vi "collectAI_img.vi"() -> (0 "wrap":i32)   [LabVIEW 2015]
uses:
  <vilib>/DAQmx/read.llb/DAQmx Read (Analog 2D I16 NChan NSamp).vi
  <vilib>/DAQmx/miscellaneous.llb/DAQmx Fill In Error Info.vi
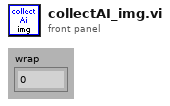
[diagram p1: front panel]
types:
  T1 = typedef "LVRectTypeDef.ctl" = cluster{"Left":i16, "Top":i16, "Right":i16, "Bottom":i16}
  T2 = cluster{"Xpixels":i32, "Vxminref":dbl, "Vxmaxref":dbl, "P":dbl, "Ypixels":i32, "Vyminref":dbl, "Vymaxref":dbl, "srate":sgl, "sAOxy":i32, "timeout":dbl, "type":string, "date":string, "time":string, "Colormap":u16, "Drawing Mode":u16, "Scanning Mode":u16, "square pixels":bool, "square matrix":bool, "Xpixels Img":i32, "Vx-min Img":dbl, "VX-max Img":dbl, "Ypixels Img":i32, "Vy-min Img":dbl, "Vy-max Img ":dbl, "Angle Img":dbl, "autoshutter":bool, "finite":bool, "cont":bool, "wavdet":bool, "measpoints":i32, "avpp":i32, "bufferAO":i32, "bufferAI":i32, "starttick":u32, "waveform":path, "Vx-ref":dbl, "Vy-ref":dbl, "refreshrate":dbl, "refreshbuffer":i32, "tt_cycles":i32, "motorref":refnum<k7>, "mirrorswitch":refnum<k7>, "sample mode":i32, "maxbufferAI":i32, "srateAODO":sgl, "bin":sgl, "Pel":sgl, "Angle draw":dbl, "srate Img":sgl, "ROIimg_plotbounds":T1, "auto OD":bool, "ODfilt":u16, "aAI":i32[], "aCI":i32[], "aAO":u32[], "aDO":u32[], "refwfsize":dbl, "Lifetime":bool, "Vz-Img":dbl, "Vz-ref":dbl, "Vz-reset":dbl, "AIoverride":bool}
  T3 = cluster{" AI":refnum<k21>, "E_AI":errorcluster, "header":dbl[]}
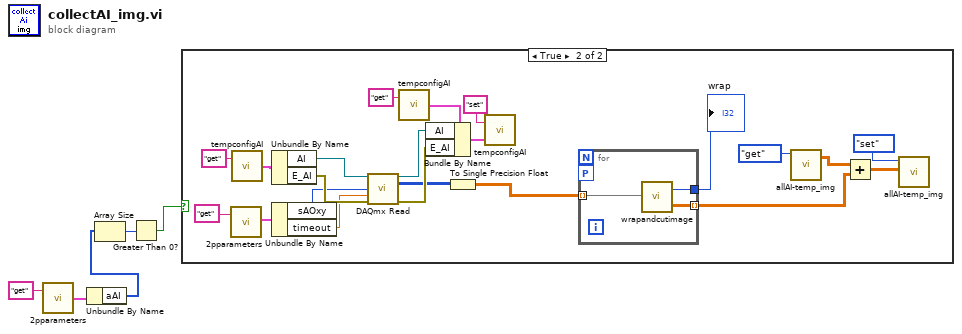
[diagram p0: block diagram]
diagram:
  n1 = call "2pparameters.vi"("command"="get") -> ("params out"=w3:T2)  [unwired: 1 in]
  n2 = Unbundle By Name(w3) -> ("aAI"=w4:i32[])
  n3 = Array Size(array=w4) -> (size(s)=w1:i32)
  n4 = Greater Than 0?(x=w1) -> (x > 0?=w5:bool)
  n5 = case shown="True" w5 {
    frame False {
    }
    frame True {
      n6 = call "2pparameters.vi"("command"="get") -> ("params out"=w14:T2)  [unwired: 1 in]
      n7 = call "tempconfigAI.vi"("command"="get") -> ("Temp Config out"=w24:T3)  [unwired: 1 in]
      n8 = Unbundle By Name(w24) -> ("AI"=w23:refnum<k21>, "E_AI"=w22:errorcluster)
      n9 = Unbundle By Name(w14) -> ("sAOxy"=w17:i32, "timeout"=w16:dbl)
      n10 = call-poly <vilib>:"DAQmx Read.vi"("task/channels in"=w23, "number of samples per channel"=w17, "timeout"=w16, "error in"=w22) -> ("task out"=w18:refnum<k21>, "data"=w13:i16[][], "error out"=w27:errorcluster)  [unwired: 9 in]
      n11 = call "tempconfigAI.vi"("command"="get") -> ("Temp Config out"=w19:T3)  [unwired: 1 in]
      n12 = Bundle By Name(cluster=w19, "AI"=w18, "E_AI"=w27) -> (w26:T3)
      n13 = To Single Precision Float(number=w13) -> (single precision float=w8:sgl[][])
      n14 = call "tempconfigAI.vi"("Temp Config in"=w26, "command"="set") -> ()  [unwired: 1 out]
      n15 = for {
        workers-P: _ -> [_]
        tunnel: w8 -> [w30] mode=indexing
        tunnel: [w29] -> w7 mode=indexing
        tunnel: [w28] -> w6
        n16 = call "wrapandcutimage.vi"("rasterscanned array"=w30) -> ("imagearray"=w29:sgl[][], "wrap"=w28:i32)
      }
      "wrap" <- w6
      n17 = call "allAI-temp_img.vi"("command"=enum16{"get", "set", "clear", "append"}."get") -> ("array out"=w11:sgl[][][])  [unwired: 3 in, 1 out]
      n18 = Add(x=w11, y=w7) -> (x+y=w12:sgl[][][])
      n19 = call "allAI-temp_img.vi"("array in"=w12, "command"=enum16{"get", "set", "clear", "append"}."set") -> ()  [unwired: 2 in, 2 out]
    }
  }
